vi "wrap angles into fitter range.vi"(10 "fit parameters":T1) -> (2 "fit parameters angles wrapped":T1)   [LabVIEW 2017]
uses:
  typedefs/magnet location fit result.ctl
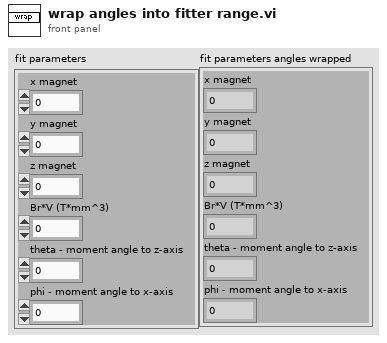
[diagram p1: front panel]
types:
  T1 = typedef "magnet location fit result.ctl" = cluster{"x magnet":dbl, "y magnet":dbl, "z magnet":dbl, "Br*V (T*mm^3)":dbl, "theta - moment angle to z-axis":dbl, "phi - moment angle to x-axis":dbl}
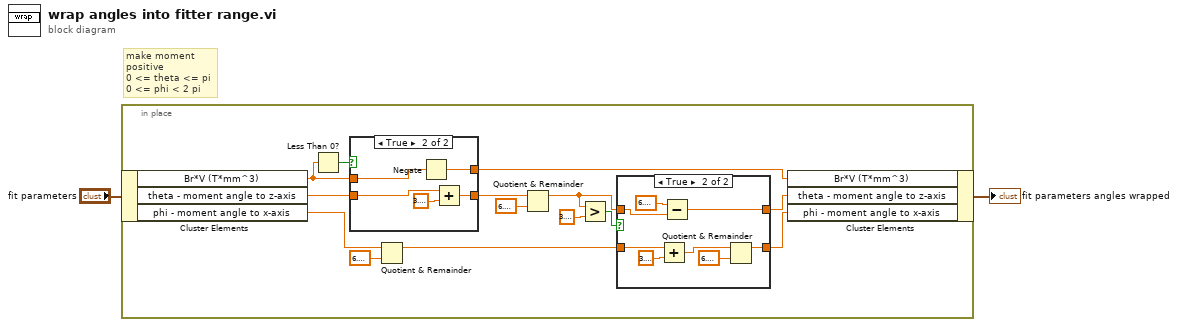
[diagram p0: block diagram]
diagram:
  # "make moment positive\n0 <= theta <= pi\n0 <= phi < 2 pi"
  n1 = in-place {
    n2 = in-place-cluster #1("fit parameters") -> ("Br*V (T*mm^3)"=w7:dbl, "theta - moment angle to z-axis"=w6:dbl, "phi - moment angle to x-axis"=w16:dbl)
    n3 = Less Than 0?(x=w7) -> (x < 0?=w8:bool)
    n4 = case shown="True" w8 {
      tunnel: w7 -> [w17 w23]
      tunnel: w6 -> [w18 w20]
      tunnel: [w18 w19] -> w5
      tunnel: [w17 w22] -> w4
      frame False {
      }
      frame True {
        n5 = Negate(x=w23) -> (-x=w22:dbl)
        n6 = Add(x=w20, y=3.141592653589793) -> (x+y=w19:dbl)
      }
    }
    n7 = Quotient & Remainder(x=w16, y=6.283185307179586) -> (x-y*floor(x/y)=w14:dbl)  [unwired: 1 out]
    n8 = Quotient & Remainder(x=w5, y=6.283185307179586) -> (x-y*floor(x/y)=w3:dbl)  [unwired: 1 out]
    n9 = Greater?(x=w3, y=3.141592653589793) -> (0:w11:bool)
    n10 = case shown="True" w11 {
      tunnel: w14 -> [w24 w33]
      tunnel: w3 -> [w25 w28]
      tunnel: [w24 w29] -> w9
      tunnel: [w25 w26] -> w10
      frame False {
      }
      frame True {
        n11 = Add(x=w33, y=3.141592653589793) -> (x+y=w31:dbl)
        n12 = Subtract(x=6.283185307179586, y=w28) -> (x-y=w26:dbl)
        n13 = Quotient & Remainder(x=w31, y=6.283185307179586) -> (x-y*floor(x/y)=w29:dbl)  [unwired: 1 out]
      }
    }
    n14 = in-place-cluster #1("Br*V (T*mm^3)"=w4, "theta - moment angle to z-axis"=w10, "phi - moment angle to x-axis"=w9) -> (→"fit parameters angles wrapped":T1)
  }
